vi "Read Sequence File.vi"(10 "Path":path) -> (1 "Test Sequence":T1[](array[typedef]), 3 "Valid?":bool)   [LabVIEW 2015]
uses:
  Single Test Sequence.ctl
  Test Sequence Action.ctl
  Valve Action Enum.ctl
  Valve Name Enum.ctl
  Test Sequence Trigger.ctl
  Sensors/Sensor Enum.ctl
  <vilib>/Utility/NIReport.llb/NI_report.lvclass
  <vilib>/addons/_office/NI_ReportGenerationToolkit.lvlib
  <vilib>/Utility/NIReport.llb/Excel/NI_Excel.lvclass
panel:
  out "error out":errorcluster
  out "current worksheet name":string
  out "worksheets count":i32
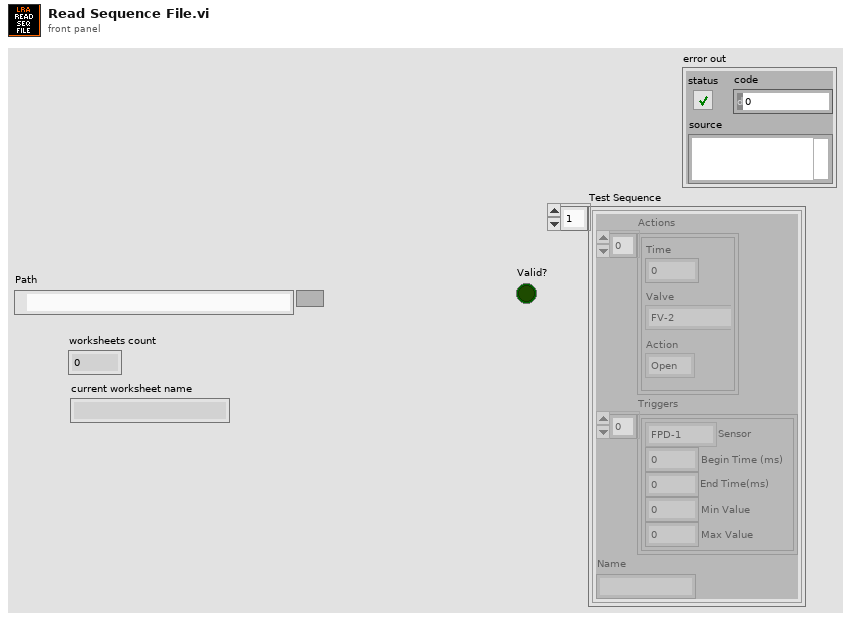
[diagram p1: front panel]
types:
  T1 = typedef "Single Test Sequence.ctl" = cluster{"Actions":T2[], "Triggers":T5[], "Name":string}
  T2 = typedef "Test Sequence Action.ctl" = cluster{"Time":i32, "Action":T3, "Valve":T4}
  T3 = typedef "Valve Action Enum.ctl" = enum16{"Open", "Close"}
  T4 = typedef "Valve Name Enum.ctl" = enum16{"FV-2", "FV-3", "FV-4", "OV-2", "OV-3", "OV-4", "COMP"}
  T5 = typedef "Test Sequence Trigger.ctl" = cluster{"Sensor":T6, "Begin Time (ms)":dbl, "End Time(ms)":dbl, "Min Value":dbl, "Max Value":dbl}
  T6 = typedef "Sensor Enum.ctl" = enum16{"FPD-1", "FPD-2", "FPD-3", "OPD-1", "OPD-2", "OPD-3", "AP-1", "VBAT", "VCOMP", "ICOMP", "TD10"}
  T7 = enum16{"Standard Report", "HTML", "Word", "Excel"}
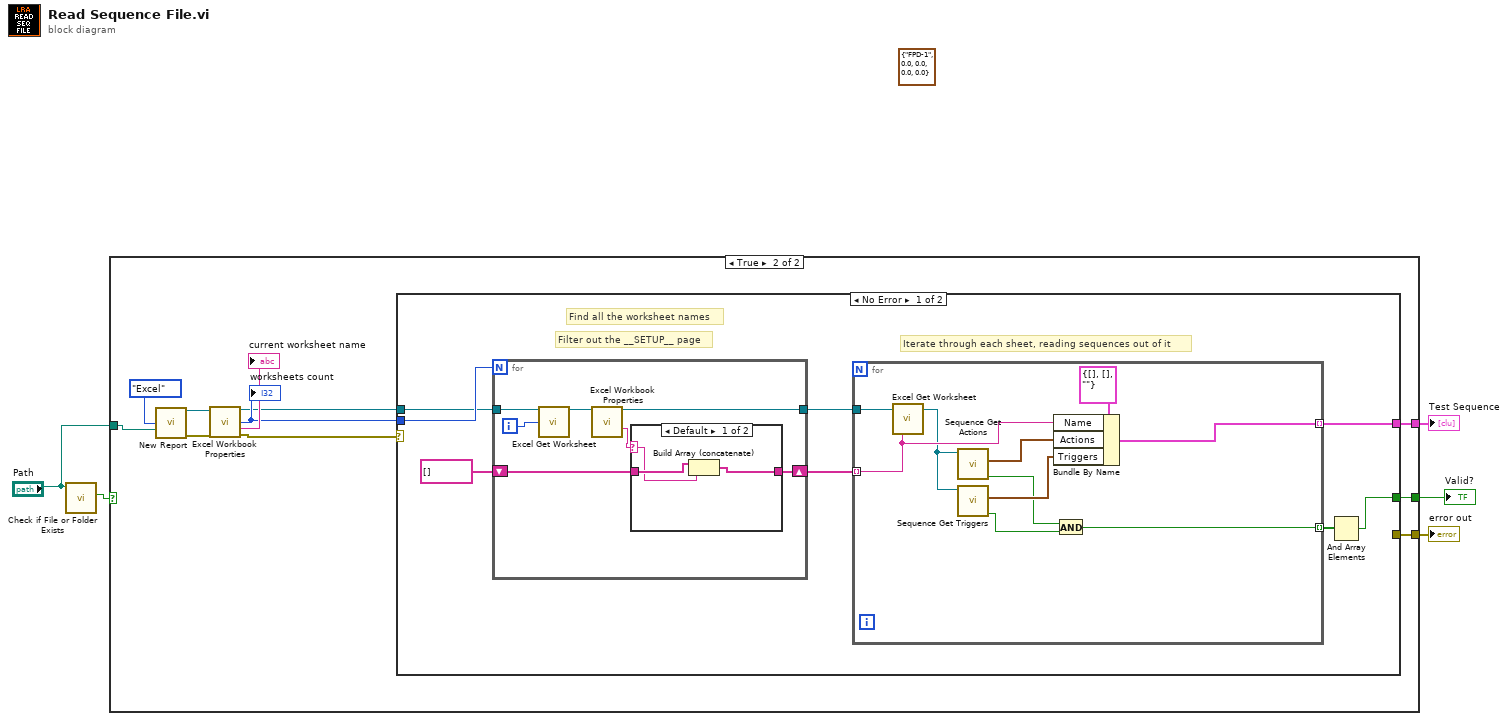
[diagram p0: block diagram]
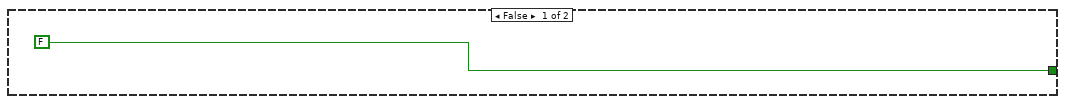
[diagram p2: hidden frame]
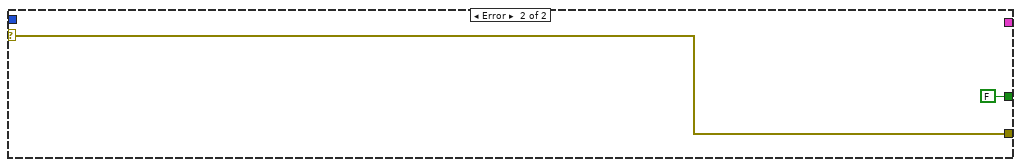
[diagram p4: hidden frame]
diagram:
  (unwired) T5 {"Sensor"=enum."FPD-1", "Begin Time (ms)"=0.0, "End Time(ms)"=0.0, "Min Value"=0.0, "Max Value"=0.0}
  n1 = call <vilib>:"Check if File or Folder Exists.vi"("path"="Path") -> ("file or folder exists?"=w5:bool)  [unwired: 8 in, 2 out]
  n2 = case shown="True" w5 {
    tunnel: [FALSE w7] -> w4
    tunnel: "Path" -> [_ w17]
    tunnel: [_ w12] -> w2
    tunnel: [_ w11] -> w1
    frame False {
    }
    frame True {
      n3 = call <vilib>:"New Report.vi"("report type"=T7."Excel", "template (empty)"=w17) -> ("report out"=w15:refnum<class "NI_report.lvclass">, "error out"=w14:errorcluster)  [unwired: 12 in]
      n4 = call <vilib>:"Excel Workbook Properties.vi"("report in"=w15, "error in (no error)"=w14) -> ("report out"=w8:refnum<class "NI_report.lvclass">, "worksheets count"=w9:i32, "current worksheet name"=→"current worksheet name":string, "error out"=w10:errorcluster)  [unwired: 10 in]
      "worksheets count" <- w9
      n5 = case shown="No Error" w10 {
        selector: w10 -> [_ w48]
        tunnel: [_ w48] -> w12
        tunnel: [w25 _] -> w11
        tunnel: w9 -> [w24 _]
        tunnel: w8 -> [w23 _]
        tunnel: [w18 FALSE] -> w7
        frame No Error {
          # "Find all the worksheet names"
          # "Filter out the __SETUP__ page"
          # "Iterate through each sheet, reading sequences out of it"
          n6 = for {
            N: w24 -> [_]
            tunnel: w23 -> [w31]
            shift-right: [w27] -> w21
            shift-left: string[] [] -> [w28]
            tunnel: [w26] -> w20
            i -> [w30]
            n7 = call <vilib>:"Excel Get Worksheet.vi"("report in"=w31, "worksheet index (0)"=w30) -> ("report out"=w32:refnum<class "NI_report.lvclass">)  [unwired: 12 in, 1 out]
            n8 = call <vilib>:"Excel Workbook Properties.vi"("report in"=w32) -> ("report out"=w26:refnum<class "NI_report.lvclass">, "current worksheet name"=w29:string)  [unwired: 11 in, 2 out]
            n9 = case shown="Default" w29 {
              selector: w29 -> [w33 _]
              tunnel: w28 -> [w34 w36]
              tunnel: [w35 w36] -> w27
              frame Default {
                n10 = Build Array (concatenate)(w34, w33) -> (w35:string[])
              }
              frame "__SETUP__" {
              }
            }
          }
          n11 = for {
            tunnel: [w45] -> w25 mode=indexing
            tunnel: w21 -> [w44] mode=indexing
            tunnel: w20 -> [w43]
            tunnel: [w37] -> w19 mode=indexing
            n12 = call <vilib>:"Excel Get Worksheet.vi"("report in"=w43, "name (\"\")"=w44) -> ("report out"=w41:refnum<class "NI_report.lvclass">)  [unwired: 12 in, 1 out]
            n13 = call "Sequence Get Actions.vi"("Excel file in"=w41) -> ("Valid?"=w39:bool, "Actions"=w42:T2[])  [unwired: 9 in]
            n14 = call "Sequence Get Triggers.vi"("Excel file in"=w41) -> ("Valid?"=w38:bool, "Triggers"=w40:T5[])  [unwired: 9 in]
            n15 = Bundle By Name(cluster=T1 {"Actions"=[], "Triggers"=[], "Name"=""} ("Cluster"), "Name"=w44, "Actions"=w42, "Triggers"=w40) -> (w45:T1)
            n16 = And(x=w39, y=w38) -> (x .and. y?=w37:bool)
          }
          n17 = And Array Elements(Boolean array=w19) -> (logical AND=w18:bool)
        }
        frame Error {
        }
      }
    }
  }
  "Valid?" <- w4
  "error out" <- w2
  "Test Sequence" <- w1
